vi "删除特定行数据.vi"(10 "目标温度":string) -> ()   [LabVIEW 2015]
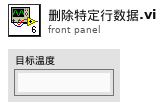
[diagram p1: front panel]
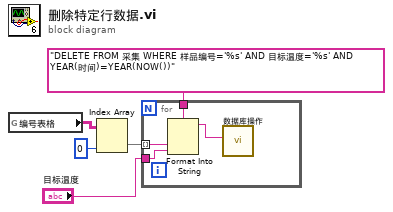
[diagram p0: block diagram]
diagram:
  n1 = global read "全局.vi" "编号表格"() -> (w4:string[][])
  n2 = Index Array(array=w4, index (col)=0 ("禁用的索引 (列)")) -> (element=w2:string[])  [unwired: 1 in]
  n3 = for {
    tunnel: w2 -> [w9] mode=indexing
    tunnel: "目标温度" -> [w8]
    tunnel: "DELETE FROM 采集 WHERE 样品编号='%s' AND 目标温度='%s' AND YEAR(时间)=YEAR(NOW())" ("SQL") -> [w7]
    n4 = Format Into String(format string=w7, w9, w8) -> (resulting string=w6:string)  [unwired: 2 in, 1 out]
    n5 = call "数据库操作.vi"("SQL query"=w6) -> ()  [unwired: 9 in, 2 out]
  }
